vi "Print AOI images.vi"(3 "Black/White Levels":cluster{ext, ext}(slide)={1.0, 65535.0} scale=1.0..65535.0, 5 "AOI Overlay?":bool=TRUE, 7 "error in (no error)":errorcluster, 8 "printer name (default)":string, 9 "Printout title":string="AOIs", 10 "Image In":T1) -> (0 "error out":errorcluster)   [LabVIEW 2011]
doc: "Make a printout of the image. Takes 8, 16, or RGB images. 8 and 16-bit images are scaled according to black/white levels and printed with aoi overlay if desired. RGB images are printed verbatim with no scaling or overlay."
uses:
  <vilib>/vision/Image Controls.llb/IMAQ Image.ctl
  <vilib>/Utility/NIReport.llb/HTML Report Image Alignment.ctl
  <vilib>/Utility/NIReport.llb/NI_report.lvclass
  <vilib>/Utility/NIReport.llb/Append Report Text (str wrap).vi
  <vilib>/Utility/NIReport.llb/Append Image to Report (string wrap).vi
  <vilib>/Utility/NIReport.llb/NI_ReportGenerationCore.lvlib
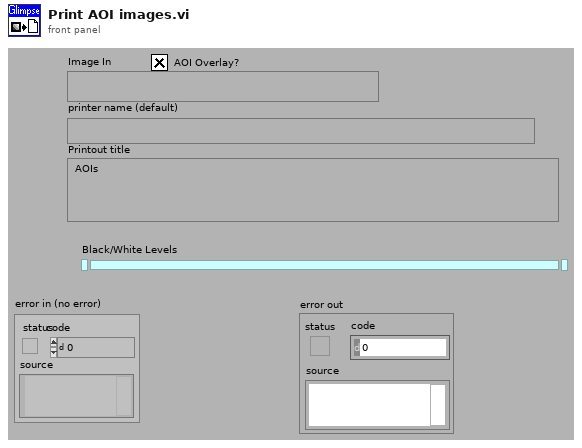
[diagram p1: front panel]
types:
  T1 = typedef "IMAQ Image.ctl" = refnum<image>
  T2 = typedef "NI_ReportGenerationCore.lvlib/HTML Report Image Alignment.ctl" = enum16{"(default)", "LEFT", "RIGHT", "TOP", "TEXTTOP", "MIDDLE", "ABSMIDDLE", "BASELINE", "BOTTOM", "ABSBOTTOM"}
  T3 = typedef "Image Type" = u32
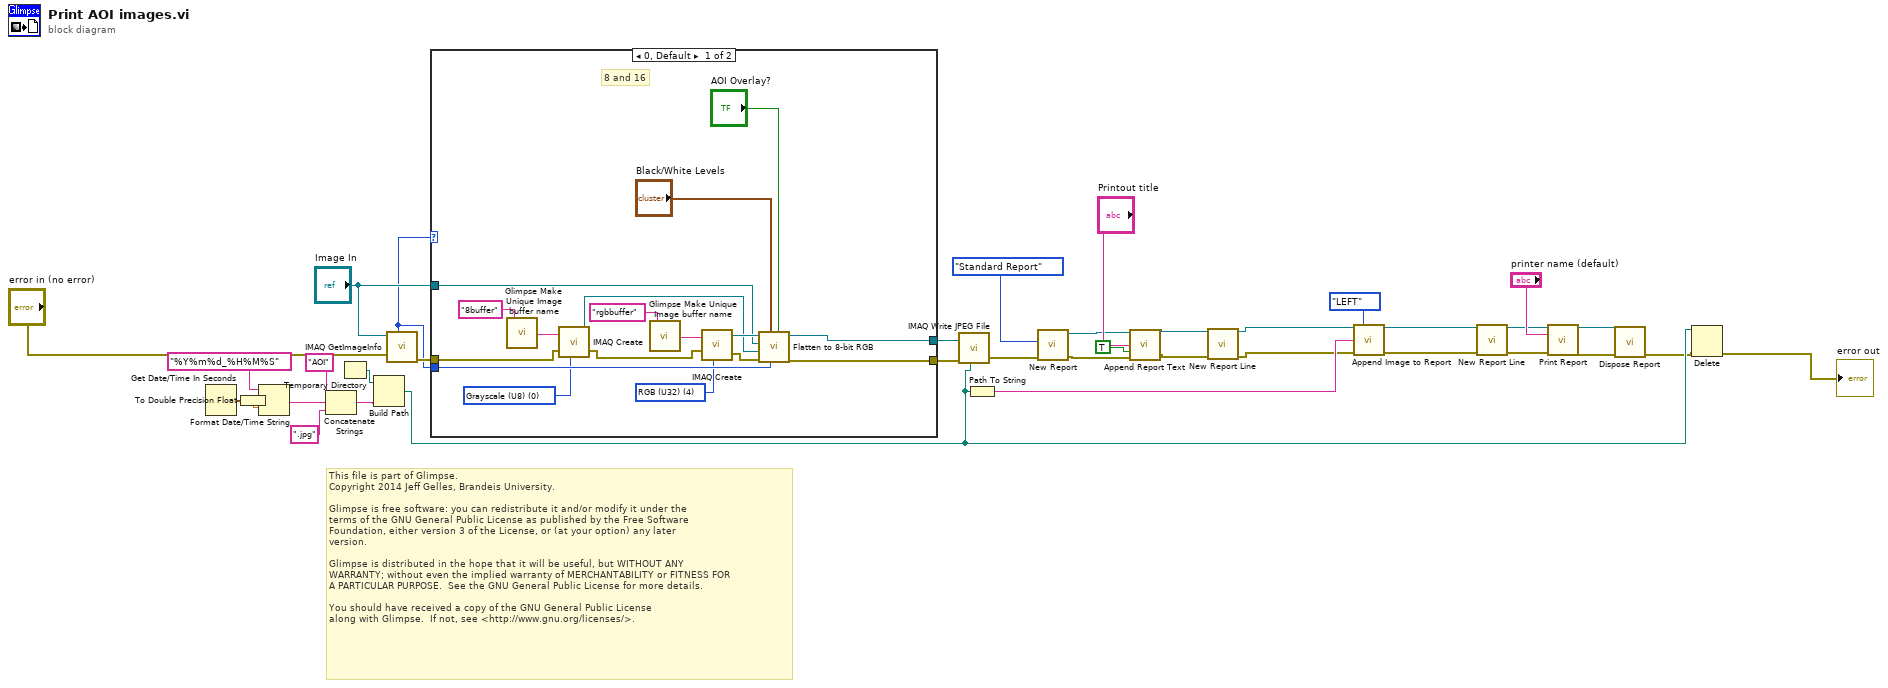
[diagram p0: block diagram]
diagram:
  # "This file is part of Glimpse. \nCopyright 2014 Jeff Gelles, Brandeis University.    \n\nGlimpse is free software: you can redistribute it and/or modify it under the \nterms of the GNU General Public License as published by the Free Software \nFoundation, either version 3 of the License, or (at your option) any later \nversion.\n\nGlimpse is distributed in the hope that it will be useful, but WITHOUT ANY \nWARRANTY; without even the implied warranty of MERCHANTABILITY or FITNESS FOR \nA PARTICULAR PURPOSE.  See the GNU General Public License for more details.\n\nYou should have received a copy of the GNU General Public License\nalong with Glimpse.  If not, see <http://www.gnu.org/licenses/>."
  n1 = Get Date/Time In Seconds() -> (seconds since 1Jan1904=w11:timestamp)
  n2 = To Double Precision Float(number=w11) -> (double precision float=w36:dbl)
  n3 = Format Date/Time String(time format string (%c)="%Y%m%d_%H%M%S", seconds (now)=w36) -> (date/time string=w27:string)  [unwired: 1 out]
  n4 = Concatenate Strings("AOI" ("string"), w27, ".jpg" ("string")) -> (w19:string)
  n5 = Temporary Directory() -> (w18:path)
  n6 = Build Path(base path=w18, name or relative path=w19) -> (appended path=w14:path)
  n7 = call "IMAQ GetImageInfo"("error in (no error)"="error in (no error)", "Image"="Image In") -> ("error out"=w7:errorcluster, "Image Type"=w6:T3)  [unwired: 8 out]
  n8 = case shown="0, Default" w6 {
    tunnel: [w49 w55] -> w10
    tunnel: [w48 w54] -> w9
    tunnel: w6 -> [w47 _]
    tunnel: "Image In" -> [w42 w55]
    tunnel: w7 -> [w41 w54]
    frame 0, Default {
      w37 = T3 4 items=["Grayscale (U8)", "Grayscale (I16)", "Grayscale (SGL)", "Complex (CSG)", "RGB (U32)", "HSL (U32)", "RGB (U64)", "Grayscale (U16)"] ("Image Type")
      w38 = T3 0 items=["Grayscale (U8)", "Grayscale (I16)", "Grayscale (SGL)", "Complex (CSG)", "RGB (U32)", "HSL (U32)", "RGB (U64)", "Grayscale (U16)"] ("Image Type")
      # "8 and 16"
      n9 = call "Glimpse Make Unique Image buffer name.vi"("Buffer  base name"="8buffer" ("Image Name")) -> ("Image Name"=w52:string)  [unwired: 1 out]
      n10 = call "IMAQ Create"("Image Name"=w52, "Image Type"=w38, "error in (no error)"=w41) -> ("New Image"=w44:T1, "error out"=w43:errorcluster)  [unwired: 1 in, 1 out]
      n11 = call "Glimpse Make Unique Image buffer name.vi"("Buffer  base name"="rgbbuffer" ("Image Name")) -> ("Image Name"=w51:string)  [unwired: 1 out]
      n12 = call "IMAQ Create"("Image Name"=w51, "Image Type"=w37, "error in (no error)"=w43) -> ("New Image"=w46:T1, "error out"=w45:errorcluster)  [unwired: 1 in, 1 out]
      n13 = call "Flatten to 8-bit RGB.vi"("AOI Overlay?"="AOI Overlay?", "Pixel depth"=w47, "Black/White Levels"="Black/White Levels", "error in"=w45, "8 bit image buffer"=w44, "8 or 16 bit image in"=w42, "RGB Image buffer"=w46) -> ("error out"=w48:errorcluster, "RGB Image Out"=w49:T1)  [unwired: 3 out]
    }
    frame 4 {
      # "RGB images are printed verbatim with no scaling or overlay"
      # "RGB"
    }
  }
  n14 = call "IMAQ Write JPEG File"("error in (no error)"=w9, "File Path"=w14, "Image"=w10) -> ("error out"=w25:errorcluster)  [unwired: 2 in, 3 out]
  n15 = Path To String(path=w14) -> (string=w17:string)
  n16 = call <vilib>:"New Report.vi"("report type"=enum16{"Standard Report", "HTML"}."Standard Report", "error in (no error)"=w25) -> ("report out"=w31:refnum<class "NI_report.lvclass">, "error out"=w30:errorcluster)  [unwired: 4 in, 8 out]
  n17 = call-poly <vilib>:"Append Report Text.vi"("report in"=w31, "text"="Printout title", "append on new line? (F)"=TRUE, "error in (no error)"=w30) -> ("report out"=w22:refnum<class "NI_report.lvclass">, "error out"=w23:errorcluster)  [unwired: 2 in, 8 out]
  n18 = call-dynamic "New Report Line.vi"("report in"=w22, "error in (no error)"=w23) -> ("report out"=w3:refnum<class "NI_report.lvclass">, "error out"=w5:errorcluster)  [unwired: 1 in, 11 out]
  n19 = call-poly <vilib>:"Append Image to Report.vi"("report in"=w3, "alignment (default)"=HTML_Report_Image_Alignment."LEFT", "path or URL of image"=w17, "error in (no error)"=w5) -> ("report out"=w2:refnum<class "NI_report.lvclass">, "error out"=w4:errorcluster)  [unwired: 2 in, 8 out]
  n20 = call-dynamic "New Report Line.vi"("report in"=w2, "error in (no error)"=w4) -> ("report out"=w16:refnum<class "NI_report.lvclass">, "error out"=w15:errorcluster)  [unwired: 1 in, 11 out]
  n21 = call-dynamic "Print Report.vi"("report in"=w16, "printer name (default)"="printer name (default)", "error in (no error)"=w15) -> ("report out"=w20:refnum<class "NI_report.lvclass">, "error out"=w24:errorcluster)  [unwired: 1 in, 10 out]
  n22 = call-dynamic "Dispose Report.vi"("report in"=w20, "error in (no error)"=w24) -> ("error out"=w13:errorcluster)  [unwired: 3 in, 10 out]
  n23 = Delete(path (use dialog)=w14, error in=w13) -> (error out=→"error out":errorcluster)  [unwired: 5 out]
